vi "get absolute position.vi"(6 "error in":errorcluster, 8 "Axis in":i32=1, 9 "VISA Handle in":refnum<visa-resource-name>) -> (0 "error out":errorcluster, 1 "Target position (units)":dbl format="%.2f", 2 "Axis out":i32=1, 3 "VISA Handle out":refnum<visa-resource-name>, 4 "TimeoutFlag":bool)   [LabVIEW 2011]
doc: "This VI returns the target position value."
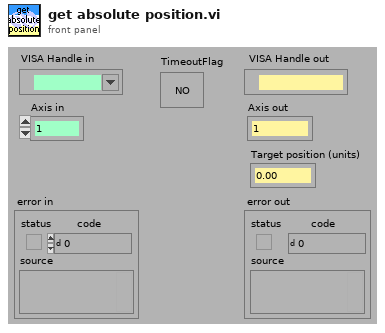
[diagram p1: front panel]
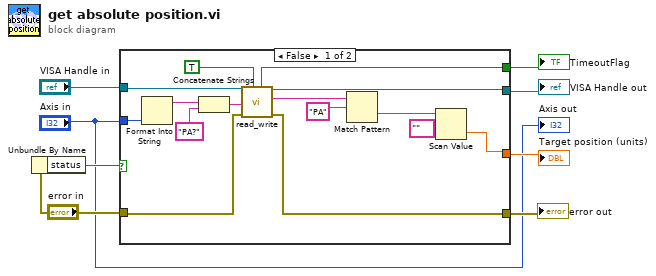
[diagram p0: block diagram]
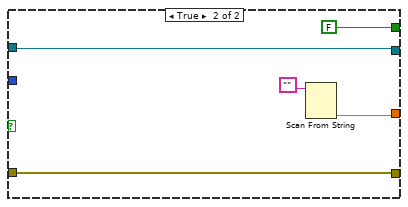
[diagram p2: hidden frame]
diagram:
  n1 = Unbundle By Name("error in") -> ("status"=w6:bool)
  n2 = case shown="False" w6 {
    tunnel: [w19 w28] -> w8
    tunnel: [w12 w25] -> w2
    tunnel: [w18 w27] -> w7
    tunnel: "VISA Handle in" -> [w22 w28]
    tunnel: "error in" -> [w20 w27]
    tunnel: [w17 FALSE ("TimeoutFlag")] -> w3
    tunnel: "Axis in" -> [w9 _]
    frame False {
      n3 = Format Into String(w9) -> (resulting string=w15:string)  [unwired: 3 in, 1 out]
      n4 = Concatenate Strings(w15, "PA?" ("string")) -> (w21:string)
      n5 = call "read_write.vi"("Query?"=TRUE, "error in"=w20, "Command"=w21, "VISA handle in"=w22) -> ("error out"=w18:errorcluster, "Response"=w14:string, "VISA handle out"=w19:refnum<visa-resource-name>, "TimeoutFlag"=w17:bool)  [unwired: 2 in]
      n6 = Match Pattern(string=w14, regular expression="PA" ("expression")) -> (after substring=w11:string)  [unwired: 1 in, 3 out]
      n7 = Scan Value(string=w11, format string="" ("chaîne de format")) -> (value=w12:dbl)  [unwired: 1 in, 1 out]
    }
    frame True {
      n8 = Scan From String(input string="") -> (output 1=w25:dbl)  [unwired: 4 in, 3 out]
    }
  }
  "VISA Handle out" <- w8
  "error out" <- w7
  "TimeoutFlag" <- w3
  "Target position (units)" <- w2
  "Axis out" <- "Axis in"
